vi "Write.vi"(8 "error in (no error)":errorcluster, 10 "Value":T1, 11 "Double Float.lvclass_340760 in":refnum<class "Var_U8.lvclass">) -> (0 "error out":errorcluster, 3 "Double Float.lvclass_340760 out":refnum<class "Var_U8.lvclass">)   [LabVIEW 2021, in "Var_U8.lvclass"]
uses:
  Var_U8.lvclass
  Type.ctl
  Var_U8.lvclass/Var_U8.ctl
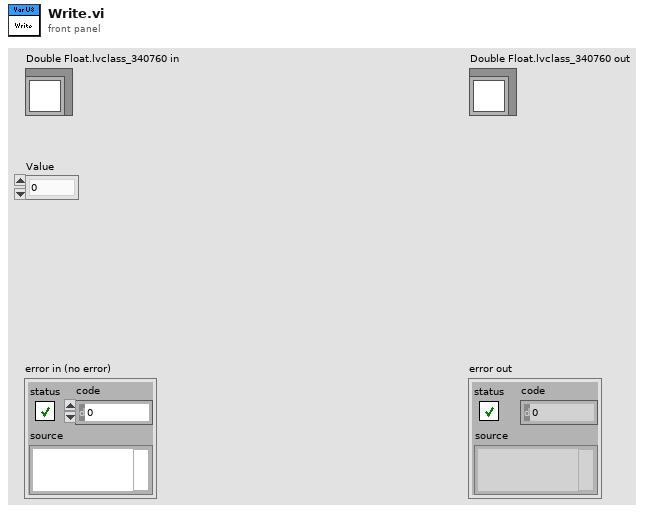
[diagram p1: front panel]
types:
  T1 = typedef "Var_U8.lvclass/Type.ctl" = u8
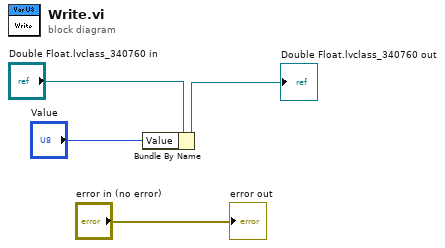
[diagram p0: block diagram]
diagram:
  n1 = Bundle By Name(cluster="Double Float.lvclass_340760 in", "Value"="Value") -> (→"Double Float.lvclass_340760 out":refnum<class "Var_U8.lvclass">)
  "error out" <- "error in (no error)"
